vi "Read Loaded Plugins.vi"(8 "error in (no error)":errorcluster, 11 "Factory Plugin Framework in":refnum<class "Factory Plugin Framework.lvclass">=refnum) -> (0 "error out":errorcluster, 2 "Loaded Plugins":T1(array[cluster]), 3 "Factory Plugin Framework out":refnum<class "Factory Plugin Framework.lvclass">)   [LabVIEW 2018, in "Factory Plugin Framework.lvlib" / "Factory Plugin Framework.lvclass"]
uses:
  Factory Plugin Framework.lvclass
  Factory Plugin Framework.lvclass/Factory Plugin Framework.ctl
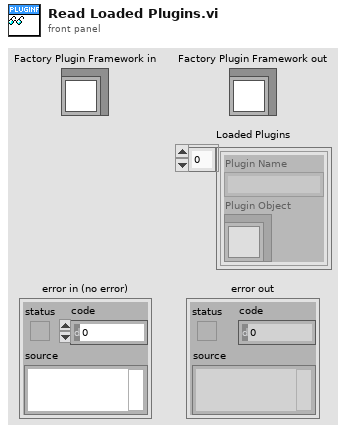
[diagram p1: front panel]
types:
  T1 = cluster{"Plugin Name":string, "Plugin Object":refnum<class>}[]
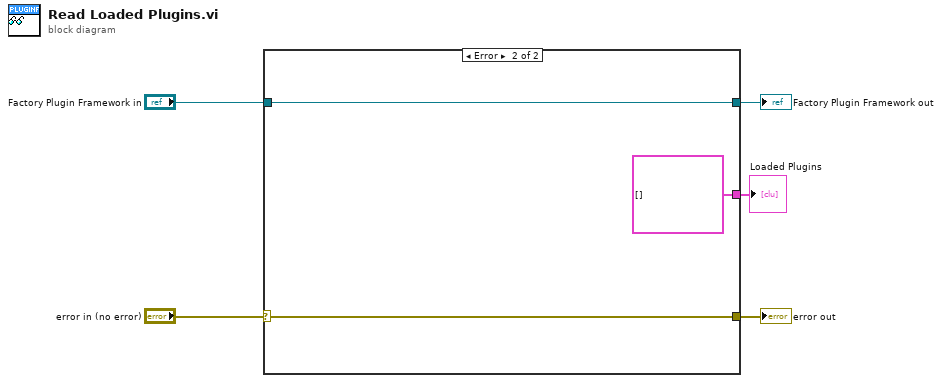
[diagram p0: block diagram]
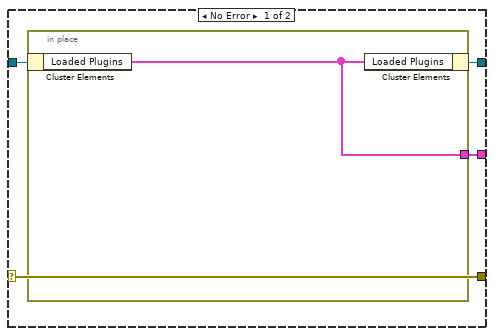
[diagram p2: hidden frame]
diagram:
  n1 = case shown="Error" "error in (no error)" {
    selector: "error in (no error)" -> [w9 w12]
    tunnel: [w9 w12] -> w4
    tunnel: [w7 w13] -> w2
    tunnel: "Factory Plugin Framework in" -> [w8 w13]
    tunnel: [w6 T1 [] ("Loaded Plugins")] -> w1
    frame No Error {
      n2 = in-place {
        in-place-border: [w10] -> w6
        n3 = in-place-cluster #1(w8) -> ("Loaded Plugins"=w10:T1)
        n4 = in-place-cluster #1("Loaded Plugins"=w10) -> (w7:refnum<class "Factory Plugin Framework.lvclass">)
      }
    }
    frame Error {
    }
  }
  "error out" <- w4
  "Factory Plugin Framework out" <- w2
  "Loaded Plugins" <- w1
